vi "AprilTag Desktop.vi"() -> ()   [LabVIEW 2025]
uses:
  filter Selector.ctl
  <vilib>/Analysis/baseanly.llb/Real Inverse Matrix.vi
  <vilib>/Analysis/NI_AALBase.lvlib
  <vilib>/vision/driver/NI_Vision_Acquisition_Software.lvlib
panel:
  in  "Hilite":bool=TRUE
  out "Instructions:":string="Run the VI using the run arrow above. Choose a camera or provided file. Update the tag family to search for.\n\nExplore and follow the AprilTag tutorial to explore accuracy and performance tradeoffs. Real-world distance and orientation measurements require tuning the scaling and intrinsic camera matrix beneath the image.\n\nThe white picture to the right is a birds-eye view of a robot with a front-facing camera. The 3D origin is shown at the top-center of the field where the apriltag is attached to that wall.  The charts farther to the right show the YPR and XYZ derived measurements in degrees and inches. Still farther is the detailed info (ID, pixel info, score, and homography matrix)."
  out "Camera IDs":string[](array[string])
  in  "Choose Camera":u16(ring) items=["FaceTime HD Camera (Built-in)  (#3E4BA11C5950E955).icd", "FaceTime HD Camera (Display)  (#BF6F5CD9C1F8410B).icd", "Microsoft® LifeCam HD-3000  (#29FE73E448C10356).icd", "Microsoft® LifeCam HD-3000  (#327B302F9406EA23).icd", "file::Tag16H5.jpg", "file::Tag36H11.jpg"]
  in  "Hamming cutoff":i32
  in  "filter":T1
  out "Y (in)":dbl format="%.1f"
  out "Z (in)":dbl format="%.1f"
  out "X (in)":dbl format="%.1f"
  in  "Length (in)":dbl=100.0
  in  "width (in)":dbl=100.0
  out "Picture":picture
  in  "show rejects":bool
  out "bad":i32
  out "loop time (s)":dbl
  in  "Scale to Inches":dbl[](array[numeric])=[2.5, 2.5, 2.5]
  out "Chart of positional info":T2(graph)
  out "YPR (deg)":cluster{"yaw":dbl, "pitch":dbl, "roll":dbl} {"yaw" format="%.1f"; "pitch" format="%.1f"; "roll" format="%.1f"}
  out "ofsets (in)":cluster{"X":dbl, "Y":dbl, "Z":dbl} {"X" format="%.1f"; "Y" format="%.1f"; "Z" format="%.1f"}
  in  "Intrinsic Camera Matrix":dbl[][](array[numeric])=[[1135.0, 0.0, 640.0], [0.0, 1135.0, 360.0], [0.0, 0.0, 1.0]]
  out "good":i32
  in  "Tag Familys":string[](array[combo])=["16h5"]
  in  "blur":dbl step=0.1
  in  "refine Edges":bool=TRUE
  in  "decimate":dbl=4.0
  in  "threads":i32=2
  out "search time (s)":dbl
  out "good tag details":T3(array[cluster])
  in  "score cutoff":dbl(slide)=60.60606060606061 scale=0.0..100.0
  out "Image":T4(plugin-control)
  # "Offset between\ntarget and camera"
  # "Angles between\ntarget and camera"
  # "Better way to pick camera matrix\ncheck other cams and simplify scaling"
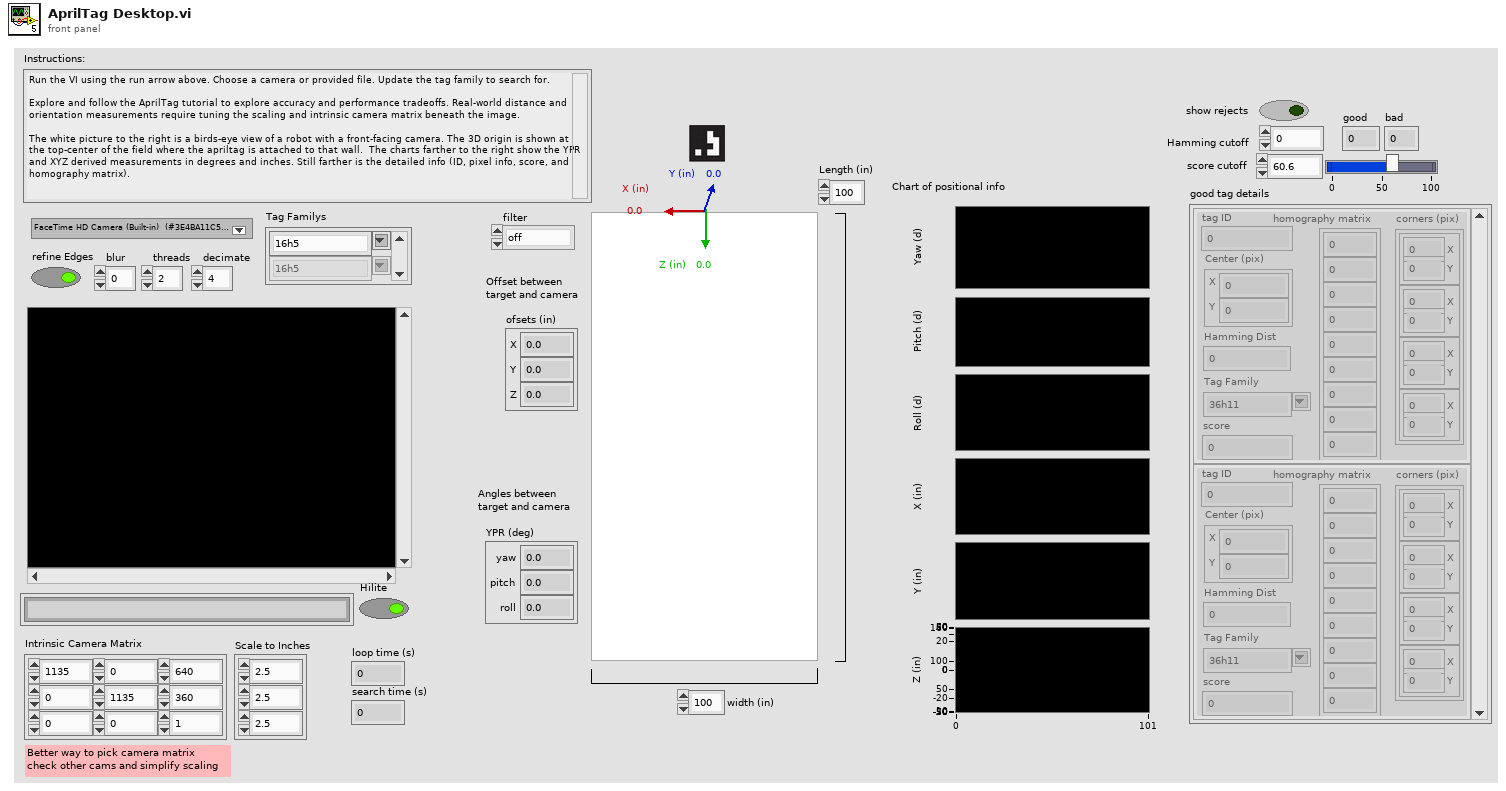
[diagram p1: front panel]
types:
  T1 = typedef "filter Selector.ctl" = enum16{"off", "2 pt avg", "low pass"}
  T2 = cluster{"yaw":dbl, "pitch":dbl, "roll":dbl, dbl, dbl, dbl}
  T3 = cluster{"tag ID":i32, "Center (pix)":cluster{"X":dbl, "Y":dbl}, "homography matrix":dbl[], "score":dbl, "Hamming Dist":i32, "corners (pix)":cluster{"X":dbl, "Y":dbl}[], "Tag Family":string}[]
  T4 = typedef "IMAQ Image.ctl" = refnum<image>
  T5 = cluster{"Type":u32, "Version":u32, "Flags":u32, "SerialNumberHigh":u32, "SerialNumberLow":u32, "BusType":u32, "InterfaceName":string, "VendorName":string, "ModelName":string, "CameraFileName":string, "CameraAttributeURL":string}[]
  T6 = typedef "Image Type" = u32
  T7 = cluster{"tag ID":i32, "Center":cluster{"X":dbl, "Y":dbl}, "homography matrix":dbl[], "decision margin":dbl, "Hamming Dist":i32, "corner points":cluster{"X":dbl, "Y":dbl}[], "Tag Family":string}[]
  T8 = cluster{"Hamming cutoff":i32, "score cutoff":dbl, "show rejects":bool}
  T9 = cluster{"tag ID":i32, "Center":cluster{"X":dbl, "Y":dbl}, "Homography Matrix":dbl[], "dec margin":dbl, "Hamming Dist":i32, "Corner Points":cluster{"X":dbl, "Y":dbl}[], "Tag Family":string}[]
  T10 = typedef "NI_Matrix.lvlib/RealMatrix.ctl" = dbl[][]
  T11 = typedef "LVBoundsTypeDef.ctl" = cluster{"Width":u32, "Height":u32}
  T12 = cluster{"tag ID":i32, "Center":cluster{"X":dbl, "Y":dbl}, "Homography Matrix":dbl[], "dec margin":dbl, "Hamming Dist":i32, "Corner Points":cluster{"X":dbl, "Y":dbl}[], "Tag Family":string}
  T13 = cluster{"Translation[0]":dbl, "Translation[1]":dbl, "Translation[2]":dbl}
  T14 = cluster{"picture out":picture, "offset":cluster{dbl, dbl}}
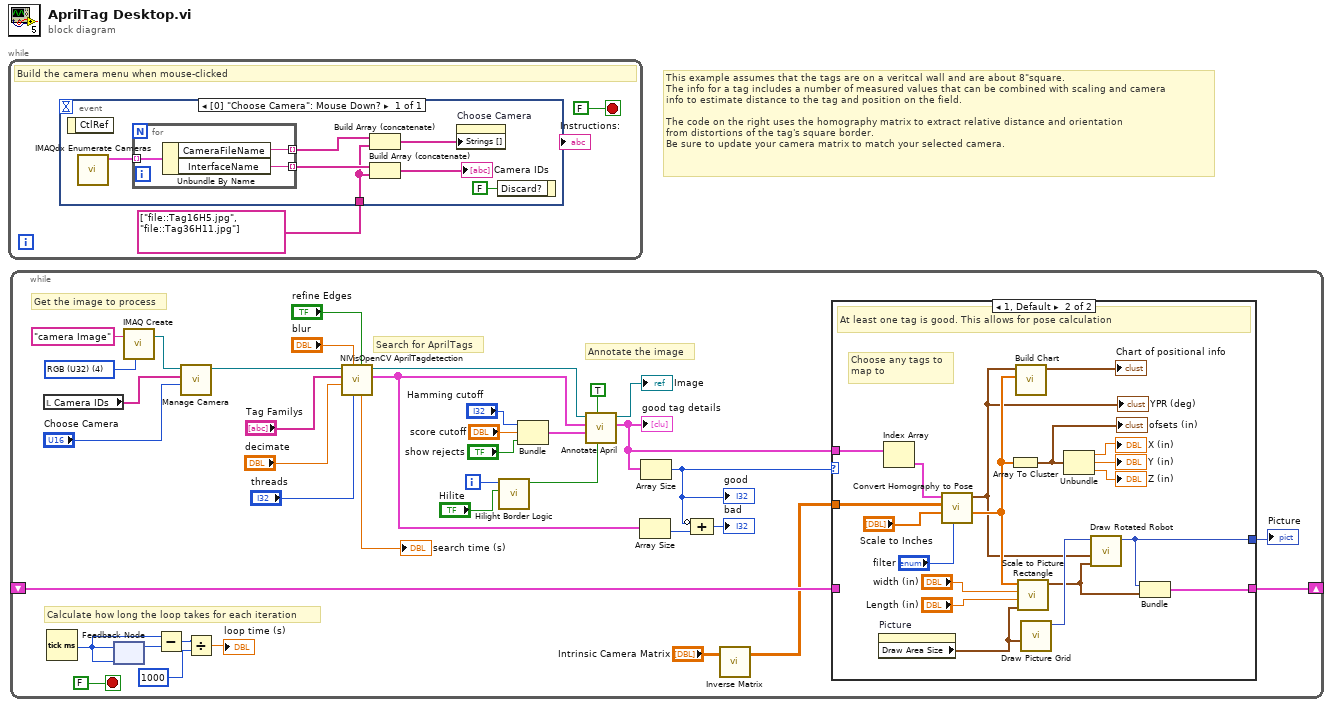
[diagram p0: block diagram]
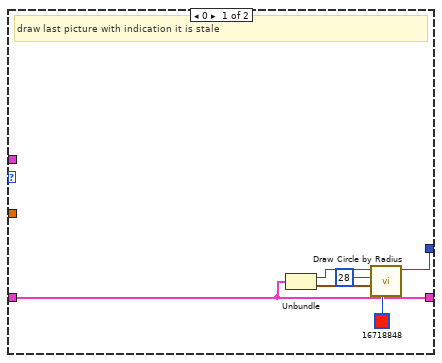
[diagram p2: hidden frame]
diagram:
  # "This example assumes that the tags are on a veritcal wall and are about 8\"square. \nThe info for a tag includes a number of measured values that can be combined with scaling and camera\ninfo to estimate distance to the tag and position on the field. \n\nThe code on the right uses the homography matrix to extract relative distance and orientation\nfrom distortions of the tag's square border.\nBe sure to update your camera matrix to match your selected camera."
  n1 = while {
    stop <- FALSE stop-if-true
    # "Build the camera menu when mouse-clicked"
    n2 = event shown="[0] \"Choose Camera\": Mouse Down?" {
      selector: _ -> [_]
      dyn-events: _ -> [_]
      timeout: _ -> [_]
      tunnel: string[] ["file::Tag16H5.jpg", "file::Tag36H11.jpg"] -> [w4]
      event "Choose Camera": Mouse Down? {
        n3 = event-data() -> ()  [unwired: 1 in, 1 out]
        n4 = call <vilib>:"IMAQdx Enumerate Cameras.vi"() -> ("Camera Information Array"=w9:T5)  [unwired: 10 in, 1 out]
        n5 = for {
          tunnel: w9 -> [w12] mode=indexing
          tunnel: [w11] -> w8 mode=indexing
          tunnel: [w10] -> w6 mode=indexing
          n6 = Unbundle By Name(w12) -> ("CameraFileName"=w11:string, "InterfaceName"=w10:string)
        }
        n7 = Build Array (concatenate)(w8, w4) -> (w7:string[])
        n8 = Build Array (concatenate)(w6, w4) -> (→"Camera IDs":string[])
        n9 = property on="Choose Camera" class="Ring (strict)"("Strings []"=w7) -> ()  [unwired: 2 in, 2 out]
        n10 = event-data("Discard?"=FALSE) -> ()  [unwired: 1 in, 1 out]
      }
    }
  }
  n11 = while {
    shift-right: [w43] -> _
    shift-left: _ -> [w44]
    i -> [w30]
    stop <- FALSE stop-if-true
    w16 = T6 4 items=["Grayscale (U8)", "Grayscale (I16)", "Grayscale (SGL)", "Complex (CSG)", "RGB (U32)", "HSL (U32)", "RGB (U64)", "Grayscale (U16)"] ("Image Type")
    # "Calculate how long the loop takes for each iteration"
    # "Annotate the image"
    # "Search for AprilTags"
    # "Get the image to process"
    n12 = local read "Camera IDs"() -> (w22:string[])
    n13 = Tick Count (ms)() -> (millisecond timer value=w41:u32)
    n14 = feedback-in #1(w41) -> ()
    n15 = feedback #1(w41) -> (w42:u32)
    n16 = call "IMAQ Create"("Image Name"="camera Image", "Image Type"=w16) -> ("New Image"=w15:T4)  [unwired: 3 in, 1 out]
    n17 = Subtract(x=w41, y=w42) -> (x-y=w33:u32)
    n18 = call "Manage Camera.vi"("Choose Camera"="Choose Camera", "Camera IDs"=w22, "Image in"=w15) -> ("Image out"=w50:T4)  [unwired: 8 in]
    n19 = Divide(x=w33, y=1000) -> (x/y=→"loop time (s)":dbl)
    n20 = call <vilib>:"NIVisOpenCV AprilTagdetection.vi"("refine Edges"="refine Edges", "threads"="threads", "blur"="blur", "decimate"="decimate", "Tag Familys"="Tag Familys", "Image Src"=w50) -> ("Detected Tags"=w24:T7, "Image Dst Out"=w49:T4, "exec time (s)"=→"search time (s)":dbl)  [unwired: 2 in, 1 out]
    n21 = call "Hilight Border Logic.vi"("Hilight"="Hilite", "index"=w30) -> ("Hilight"=w29:bool)  [unwired: 9 in]
    n22 = Bundle("Hamming cutoff"="Hamming cutoff", "score cutoff"="score cutoff", "show rejects"="show rejects") -> (w25:T8)  [unwired: 1 in]
    n23 = call "Annotate April.vi"("hilight"=w29, "Annotate"=TRUE ("Show displays"), "cutoffs"=w25, "Detected Tags"=w24, "Refnum in"=w49) -> ("tags"=w23:T9, "Refnum out"=→"Image":T4)  [unwired: 4 in, 1 out]
    "good tag details" <- w23
    n24 = Array Size(array=w24) -> (size(s)=w40:i32)
    n25 = Array Size(array=w23) -> (size(s)=w20:i32)
    "good" <- w20
    n26 = Compound Arithmetic op=ADD(invert w20, w40) -> (→"bad":i32)
    n27 = call-poly <vilib>:"Inverse Matrix.vi"("Input Matrix"="Intrinsic Camera Matrix") -> ("Inverse Matrix"=w18:T10)  [unwired: 1 in, 1 out]
    n28 = case shown="1, Default" w20 {
      tunnel: w18 -> [_ w75]
      tunnel: [w56 w71] -> w45
      tunnel: w44 -> [w51 _]
      tunnel: [w51 w70] -> w43
      tunnel: w23 -> [_ w69]
      frame 0 {
        # "draw last picture with indication it is stale"
        n29 = Unbundle(w51) -> ("picture out"=w55:picture, "offset"=w54:cluster{dbl, dbl})
        n30 = call <vilib>:"Draw Circle by Radius.vi"("color(black)"=u32 16718848, "pixel center"=w54, "radius"=i16 28, "picture"=w55) -> ("new picture"=w56:picture)  [unwired: 7 in]
      }
      frame 1, Default {
        # "Choose any tags to\nmap to"
        # "At least one tag is good. This allows for pose calculation"
        n31 = property on="Picture" class="Pict"() -> ("Draw Area Size"=w60:T11)  [unwired: 2 in, 2 out]
        n32 = Index Array(array=w69) -> (element=w59:T12)  [unwired: 1 in]
        n33 = call "Convert Homography to Pose.vi"("filter"="filter", "Scale to Inches"="Scale to Inches", "Inverse Camera Matrix"=w75, "tag info"=w59) -> ("Translation"=w61:dbl[], "angles (deg)"=w58:cluster{"yaw":dbl, "pitch":dbl, "roll":dbl})  [unwired: 5 in, 1 out]
        "YPR (deg)" <- w58
        n34 = Array To Cluster(array=w61) -> (cluster=w62:T13)
        "ofsets (in)" <- w62
        n35 = call "Build Chart.vi"("Translation"=w61, "angles (deg)"=w58) -> ("chart data"=→"Chart of positional info":T2)  [unwired: 9 in]
        n36 = call "Scale to Picture Rectangle.vi"("Draw Area Size"=w60, "Length (in)"="Length (in)", "width (in)"="width (in)", "Translation XYZ"=w61) -> ("offset"=w66:cluster{dbl, dbl})  [unwired: 7 in]
        n37 = call "Draw Picture Grid.vi"("Draw Area Size"=w60) -> ("picture out"=w68:picture)  [unwired: 10 in]
        n38 = Unbundle(w62) -> ("Translation[0]"=→"X (in)":dbl, "Translation[1]"=→"Y (in)":dbl, "Translation[2]"=→"Z (in)":dbl)
        n39 = call "Draw Rotated Robot.vi"("offset"=w66, "YPR (deg)"=w58, "Picture in"=w68) -> ("picture out"=w71:picture)  [unwired: 8 in]
        n40 = Bundle("picture out"=w71, "offset"=w66) -> (w70:T14)  [unwired: 1 in]
      }
    }
    "Picture" <- w45
  }
